vi "Create TDMS File.vi"(8 "error in":errorcluster, 10 "Active Modules":string[](array[string]), 11 "file path":path) -> (0 "error out":errorcluster, 3 "tdms file out":refnum<k34>)   [LabVIEW 2024, in "Thermal Chamber.lvlib"]
doc: "<b>Note:</b> This VI was modified by the <b>Validate DQMH Module</b> tool to be shared clone reentrant."
uses:
  Thermal Chamber.lvlib
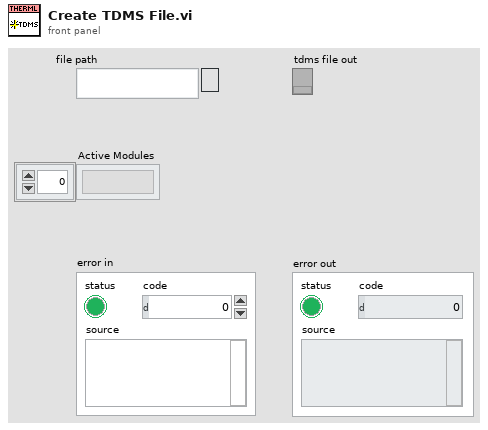
[diagram p1: front panel]
types:
  T1 = enum16{"open", "open or create", "create or replace", "create", "open (read-only)"}
  T2 = cluster{"Group Name":string, "Channel Name":string, "Units":string, "Sample Rate (Hz)":dbl}[]
  T3 = cluster{"Group Name":string, "Channel Name":string, "Units":string, "Sample Rate (Hz)":dbl}
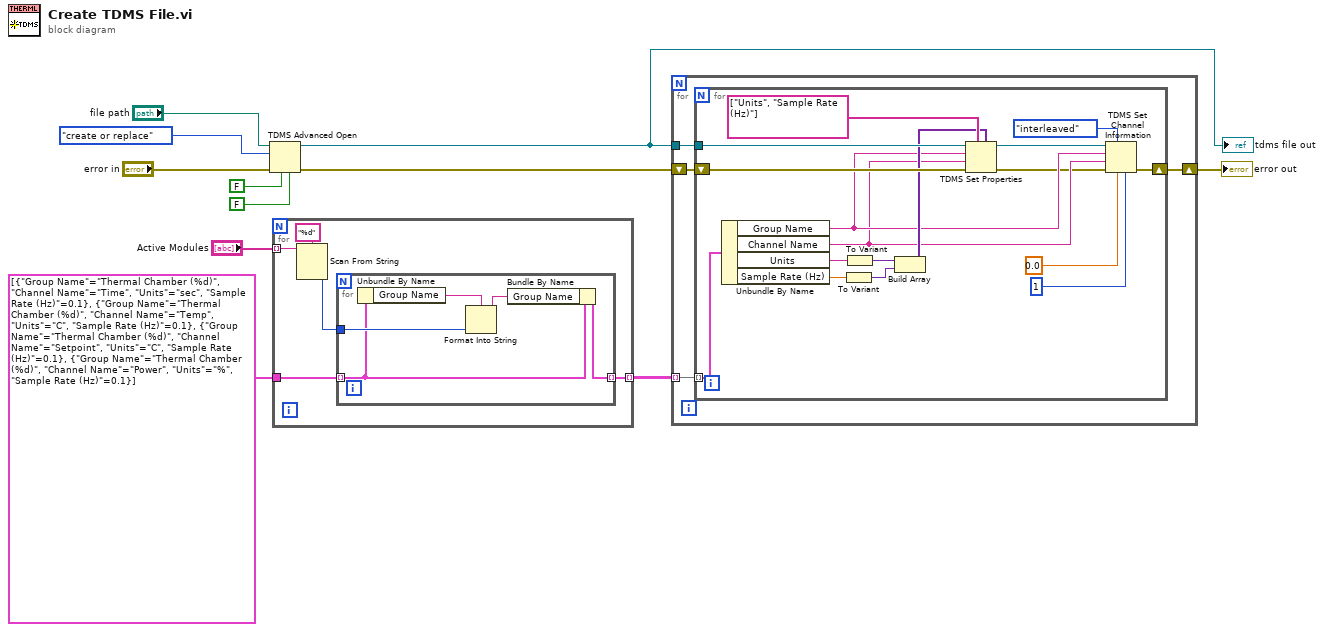
[diagram p0: block diagram]
diagram:
  n1 = TDMS Advanced Open(4:FALSE ("enable asynchronous? (T)"), 6:FALSE ("disable buffering? (T)"), 8:"error in", 10:T1."create or replace" ("operation (0:open)"), 11:"file path") -> (0:w6:errorcluster, 3:w1:refnum<k34>)  [unwired: 1 out]
  "tdms file out" <- w1
  n2 = for {
    tunnel: "Active Modules" -> [w15] mode=indexing
    tunnel: T2 [{"Group Name"="Thermal Chamber (%d)", "Channel Name"="Time", "Units"="sec", "Sample Rate (Hz)"=0.1}, {"Group Name"="Thermal Chamber (%d)", "Channel Name"="Temp", "Units"="C", "Sample Rate (Hz)"=0.1}, {"Group Name"="Thermal Chamber (%d)", "Channel Name"="Setpoint", "Units"="C", "Sample Rate (Hz)"=0.1}, {"Group Name"="Thermal Chamber (%d)", "Channel Name"="Power", "Units"="%", "Sample Rate (Hz)"=0.1}] -> [w13]
    tunnel: [w12] -> w5 mode=indexing
    n3 = Scan From String(format string="%d", input string=w15) -> (output 1=w14:i32)  [unwired: 3 in, 3 out]
    n4 = for {
      tunnel: w14 -> [w20]
      tunnel: w13 -> [w19] mode=indexing
      tunnel: [w18] -> w12 mode=indexing
      n5 = Unbundle By Name(w19) -> ("Group Name"=w21:string)
      n6 = Format Into String(format string=w21, w20) -> (resulting string=w17:string)  [unwired: 2 in, 1 out]
      n7 = Bundle By Name(cluster=w19, "Group Name"=w17) -> (w18:T3)
    }
  }
  n8 = for {
    tunnel: w1 -> [w24]
    tunnel: w5 -> [w23] mode=indexing
    shift-right: [w22] -> w4
    shift-left: w6 -> [w25]
    n9 = for {
      tunnel: w23 -> [w36] mode=indexing
      shift-right: [w26] -> w22
      shift-left: w25 -> [w39]
      tunnel: w24 -> [w38]
      n10 = Unbundle By Name(w36) -> ("Group Name"=w30:string, "Channel Name"=w29:string, "Units"=w35:string, "Sample Rate (Hz)"=w34:dbl)
      n11 = To Variant(anything=w34) -> (Variant=w32:variant)
      n12 = To Variant(anything=w35) -> (Variant=w33:variant)
      n13 = Build Array(w33, w32) -> (w31:variant[])
      n14 = TDMS Set Properties(5:w31, 7:string[] ["Units", "Sample Rate (Hz)"], 8:w39, 9:w29, 10:w30, 11:w38) -> (0:w28:errorcluster, 3:w27:refnum<k34>)  [unwired: 2 out]
      n15 = TDMS Set Channel Information(4:u32 1 ("samples per channel"), 6:0.0, 7:enum16{"non-interleaved", "interleaved"}."interleaved" ("data layout (0:non-interleaved)"), 8:w28, 9:w29, 10:w30, 11:w27) -> (0:w26:errorcluster)  [unwired: 1 out]
    }
  }
  "error out" <- w4
